vi "Status Mode.vi"(7 "Detailed Information (F)":bool, 8 "error in (no error)":errorcluster, 10 "Address (0)":i32, 11 "VISA resource name":refnum<visa-resource-name>) -> (0 "error out":errorcluster, 2 "MODE":T1=enum."OFF", 3 "VISA resource name out":refnum<visa-resource-name>)   [LabVIEW 2016, in "Environment Chamber.lvlib" / "Climatic Chamber.lvlib"]
doc: "<b>Operation mode monitor</B>\n\nReturns the (detailed) chamber operation state.\n\n<b>Standard information:</B>\n- OFF\n- STANDBY\n- CONSTANT\n- RUN\n\n<b>Detailed information:</B>\n- OFF\n- STANDBY\n- CONSTANT\n- RUN\n- RUN PAUSE\n- RUN END HOLD\n- RMT RUN\n- RMT RUN PAUSE\n- RMT RUN END HOLD"
uses:
  Climatic Chamber.lvlib
  Private/Type Defs/Mode Enum.ctl
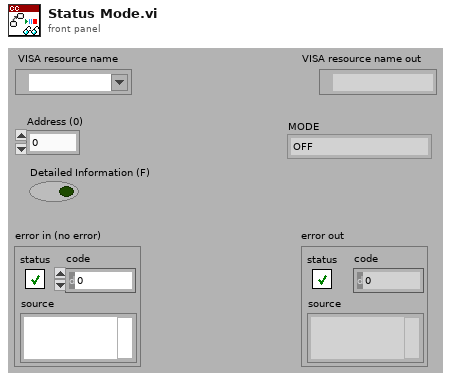
[diagram p1: front panel]
types:
  T1 = typedef "Environment Chamber.lvlib/Climatic Chamber.lvlib/Mode Enum.ctl" = enum16{"ERROR", "OFF", "STANDBY", "CONSTANT", "RUN", "RUN PAUSE", "RUN END HOLD", "RMT RUN", "RMT RUN PAUSE", "RMT RUN END HOLD"}
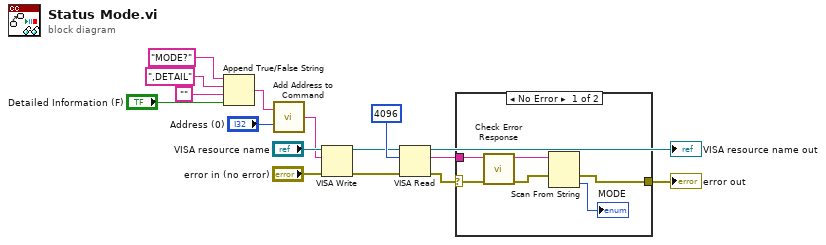
[diagram p0: block diagram]
diagram:
  n1 = Append True/False String(1:"Detailed Information (F)", 2:"", 3:",DETAIL", 4:"MODE?" ("string (\"\")")) -> (0:w2:string)
  n2 = call "Add Address to Command.vi"("Address (0)"="Address (0)", "Command"=w2) -> ("Command OUT"=w9:string)
  n3 = VISA Write(VISA resource name="VISA resource name", write buffer=w9, error in (no error)="error in (no error)") -> (VISA resource name out=w13:refnum<visa-resource-name>, error out=w12:errorcluster)  [unwired: 1 out]
  n4 = VISA Read(VISA resource name=w13, byte count=u32 4096, error in (no error)=w12) -> (VISA resource name out=→"VISA resource name out":refnum<visa-resource-name>, read buffer=w7:string, error out=w8:errorcluster)  [unwired: 1 out]
  n5 = case shown="No Error" w8 {
    selector: w8 -> [w20 w23]
    tunnel: w7 -> [w21 _]
    tunnel: [w22 w23] -> w6
    frame No Error {
      n6 = call "Check Error Response.vi"("error in (no error)"=w20, "read String"=w21) -> ("error out"=w17:errorcluster, "String out"=w19:string)  [unwired: 7 in, 1 out]
      n7 = Scan From String(input string=w19, error in=w17) -> (error out=w22:errorcluster, output 1=→"MODE":T1)  [unwired: 3 in, 2 out]
    }
    frame Error {
    }
  }
  "error out" <- w6
